vi "Set Address.vi"(6 "chip select  (1st chip)":enum16{"1st chip", "2nd chip"}(ring), 8 "error in (no error)":errorcluster, 9 "address":u8 format="%.0x", 10 "address type (DDRAM)":enum16{"DDRAM", "CGRAM"}(ring), 11 "LCD in":refnum<class "Character LCD.lvclass">) -> (0 "error out":errorcluster, 3 "LCD out":refnum<class "Character LCD.lvclass">)   [LabVIEW 2015, in "HD44780 Host.lvlib"]
uses:
  HD44780 Host.lvlib
  Internal/LCD Class/Character LCD.lvclass
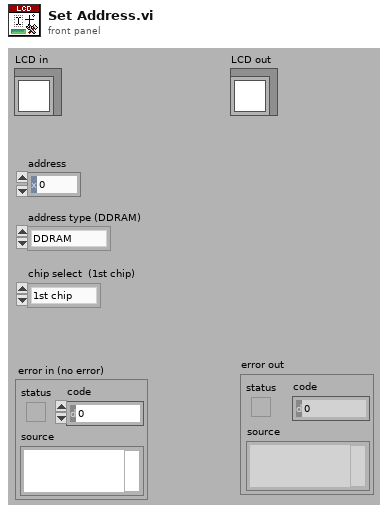
[diagram p1: front panel]
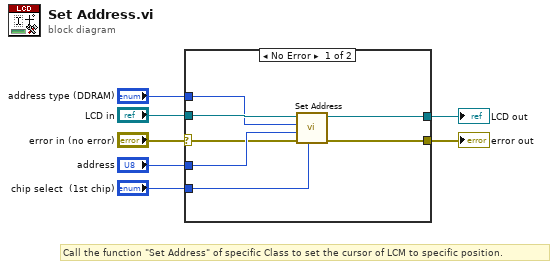
[diagram p0: block diagram]
diagram:
  # "Call the function \"Set Address\" of specific Class to set the cursor of LCM to specific position."
  n1 = case shown="No Error" "error in (no error)" {
    selector: "error in (no error)" -> [w9 w16]
    tunnel: "address" -> [w14 _]
    tunnel: "address type (DDRAM)" -> [w8 _]
    tunnel: "chip select  (1st chip)" -> [w13 _]
    tunnel: [w11 w16] -> w4
    tunnel: "LCD in" -> [w12 w15]
    tunnel: [w10 w15] -> w1
    frame No Error {
      n2 = call-dynamic "Set Address.vi"("chip select  (1st chip)"=w13, "error in (no error)"=w9, "address"=w14, "address type (DDRAM)"=w8, "Character LCD in"=w12) -> ("error out"=w11:errorcluster, "Character LCD out"=w10:refnum<class "Character LCD.lvclass">)  [unwired: 5 in]
    }
    frame Error {
    }
  }
  "error out" <- w4
  "LCD out" <- w1
